vi "main(Test DQMH modules).bak.vi"() -> ()   [LabVIEW 2018, in "Application.lvlib"] (continued)
    "DC Measure Completed" <- w229
    "Progress" <- w226
    n4221 = feedback-in #1(w226) -> ()
    n4222 = disable-structure shown="LOGGING==TRUE" {
      disable-tunnel: [w253 _] -> w227
      disable-tunnel: w228 -> [w250 _]
      frame condition #0 (active) {
        n4223 = property on="State log" class="Str"("Text.Scroll Position"=inf) -> ()  [unwired: 2 in, 2 out]
        n4224 = call "string log (SubVI).vi"("error in (no error)"=w250, "Enum"=enum16{"Init", "Log", "Read"}."Read") -> ("error out"=w253:errorcluster, "State log"=→"State log":string)  [unwired: 8 in]
      }
      frame condition #1 {
      }
    }
  }
  n4225 = Unregister For Events(event registration refnum=w94) -> (error out=w10:errorcluster)  [unwired: 1 in]
  n4226 = Release Queue(queue=w90, error in (no error)=w89) -> (error out=w8:errorcluster)  [unwired: 1 in, 2 out]
  n4227 = Destroy User Event(user event=w7, error in=w8) -> (error out=w4:errorcluster)
  n4228 = while {
    shift-right: [w9129] -> w3
    shift-left: w5 -> [w9131]
    shift-right: [w9126] -> w2
    shift-left: w4 -> [w9130]
    stop <- w9127 stop-if-true
    n4229 = Get Queue Status(queue=w9131, error in (no error)=w9130) -> (queue out=w9129:refnum<queue>, error out=w9126:errorcluster, # elements in queue=w9128:i32)  [unwired: 1 in, 5 out]
    n4230 = Equal To 0?(x=w9128) -> (x = 0?=w9127:bool)
    n4231 = Wait (ms)(milliseconds to wait=u32 10) -> ()  [unwired: 1 out]
  }
  n4232 = Release Queue(queue=w3, error in (no error)=w2) -> (error out=w1:errorcluster)  [unwired: 1 in, 2 out]
  n4233 = Merge Errors(w10, w1) -> (w9:errorcluster)
  n4234 = disable-structure shown="RUN_TIME_ENGINE==True" {
    disable-tunnel: w9 -> [w9132 _]
    frame condition #0 (active) {
      "error out" <- w9132
    }
    frame condition #1 {
      n4235 = Quit LabVIEW(quit? (T)=TRUE) -> ()
    }
  }
